vi "json token return after.vi"(9 "string index":i32, 10 "token in":i32, 11 "tokens in":T1[](array[typedef])) -> (2 "token out":i32, 3 "tokens out":T1[](array[typedef]))   [LabVIEW 2013]
uses:
  json token.ctl
  json node type.ctl
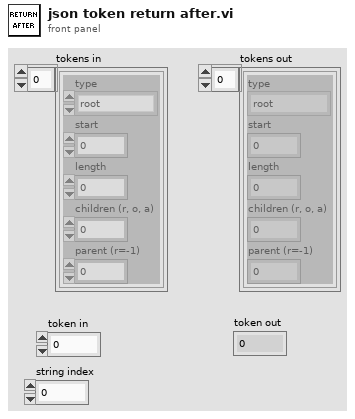
[diagram p1: front panel]
types:
  T1 = typedef "json token.ctl" = cluster{"type":T2, "start":i32, "length":i32, "children (r, o, a)":u16, "parent (r=-1)":i32}
  T2 = typedef "json node type.ctl" = enum16{"root", "object", "array", "number", "string value", "string key", "true", "false", "null"}
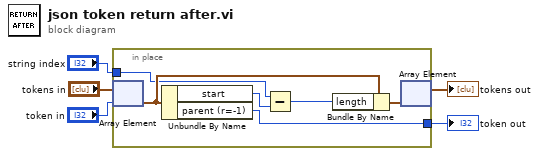
[diagram p0: block diagram]
diagram:
  n1 = in-place {
    in-place-border: [w11] -> w2
    in-place-border: "string index" -> [w7]
    n2 = in-place-array #1("tokens in", "token in") -> (w10:T1)
    n3 = Unbundle By Name(w10) -> ("start"=w6:i32, "parent (r=-1)"=w11:i32)
    n4 = Subtract(x=w7, y=w6) -> (x-y=w8:i32)
    n5 = Bundle By Name(cluster=w10, "length"=w8) -> (w9:T1)
    n6 = in-place-array #1(w9) -> (→"tokens out":T1[])  [unwired: 1 out]
  }
  "token out" <- w2
